vi "AprilTagFieldLayout_New2022.vi"() -> (3 "AprilTagFieldLayout":T1={"AprilTagMap"={}, "FieldLength"=0.0, "FieldWidth"=0.0, "OriginPosition "=enum."kBlueAllianceWallRightSide,", "OriginPose3d"={"Translation3d"={"X"=0.0, "Y"=0.0, "Z"=0.0}, "Rotation3d"={"Q_quaternion"={"R"=1.0, "V"=[0.0, 0.0, 0.0]}}}} {"OriginPose3d"."Translation3d"."Z" format="%14.3f"; "OriginPose3d"."Translation3d"."Y" format="%14.3f"; "OriginPose3d"."Translation3d"."X" format="%14.3f"})   [LabVIEW 2019, in "Trajectory_Library.lvlib"]
doc: "Define the FRC 2022 April Tag field layout.\n\nNOTE -- This function has not been completed.\n\nInputs:\n <none>\n\nOutputs:\n -- AprilTagFieldLayout -- AprilTagFieldLayout -- Data cluster containing field definition."
uses:
  Trajectory_Library.lvlib
  TypeDef/AprilTagFieldLayout.ctl
  TypeDef/AprilTag.ctl
  TypeDef/POSE3D.ctl
  TypeDef/TRANSLATION3D.ctl
  TypeDef/ROTATION3D.ctl
  TypeDef/QUATERNION.ctl
  Enum/AprilTagFieldLayoutOrignPosition_ENUM.ctl
  AprilTag_GetAll.vi
  Quaternion_Normalize.vi
  Quaternion_New_Default.vi
panel:
  # "NOT DONE"
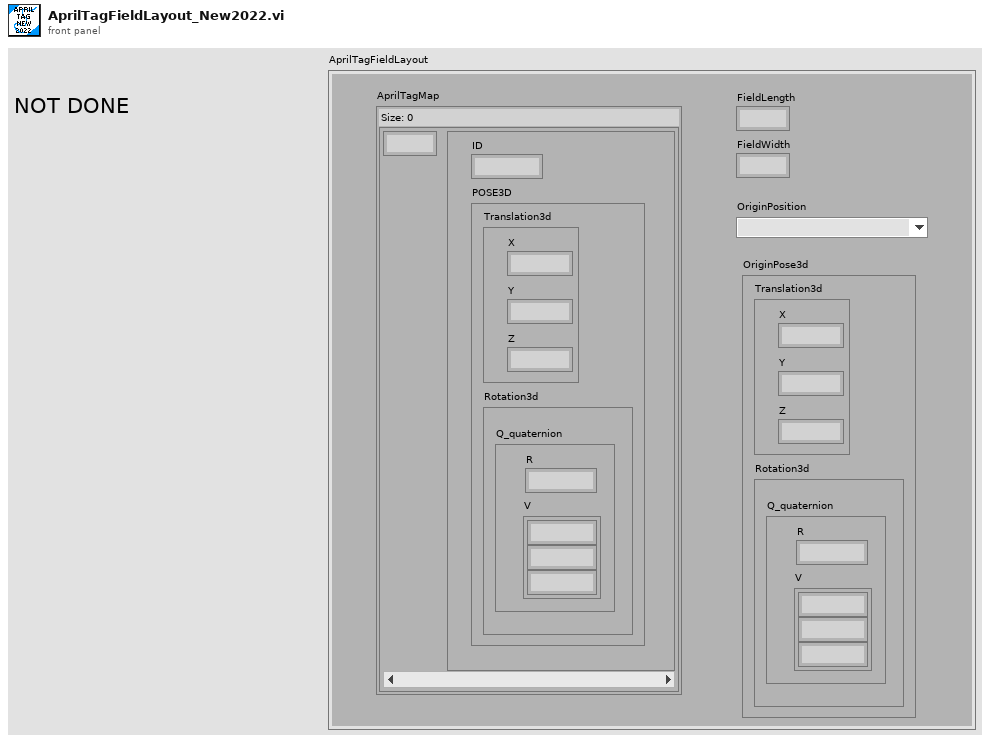
[diagram p1: front panel]
types:
  T1 = typedef "Trajectory_Library.lvlib/AprilTagFieldLayout.ctl" = cluster{"AprilTagMap":map{i32, T2}, "FieldLength":dbl, "FieldWidth":dbl, "OriginPosition ":T7, "OriginPose3d":T3}
  T2 = typedef "Trajectory_Library.lvlib/AprilTag.ctl" = cluster{"ID":i32, "POSE3D":T3}
  T3 = typedef "Trajectory_Library.lvlib/POSE3D.ctl" = cluster{"Translation3d":T4, "Rotation3d":T5}
  T4 = typedef "Trajectory_Library.lvlib/TRANSLATION3D.ctl" = cluster{"X":dbl, "Y":dbl, "Z":dbl}
  T5 = typedef "Trajectory_Library.lvlib/ROTATION3D.ctl" = cluster{"Q_quaternion":T6}
  T6 = typedef "Trajectory_Library.lvlib/QUATERNION.ctl" = cluster{"R":dbl, "V":dbl[]}
  T7 = typedef "Trajectory_Library.lvlib/AprilTagFieldLayoutOrignPosition_ENUM.ctl" = enum16{"kBlueAllianceWallRightSide,", "kRedAllianceWallRightSide,"}
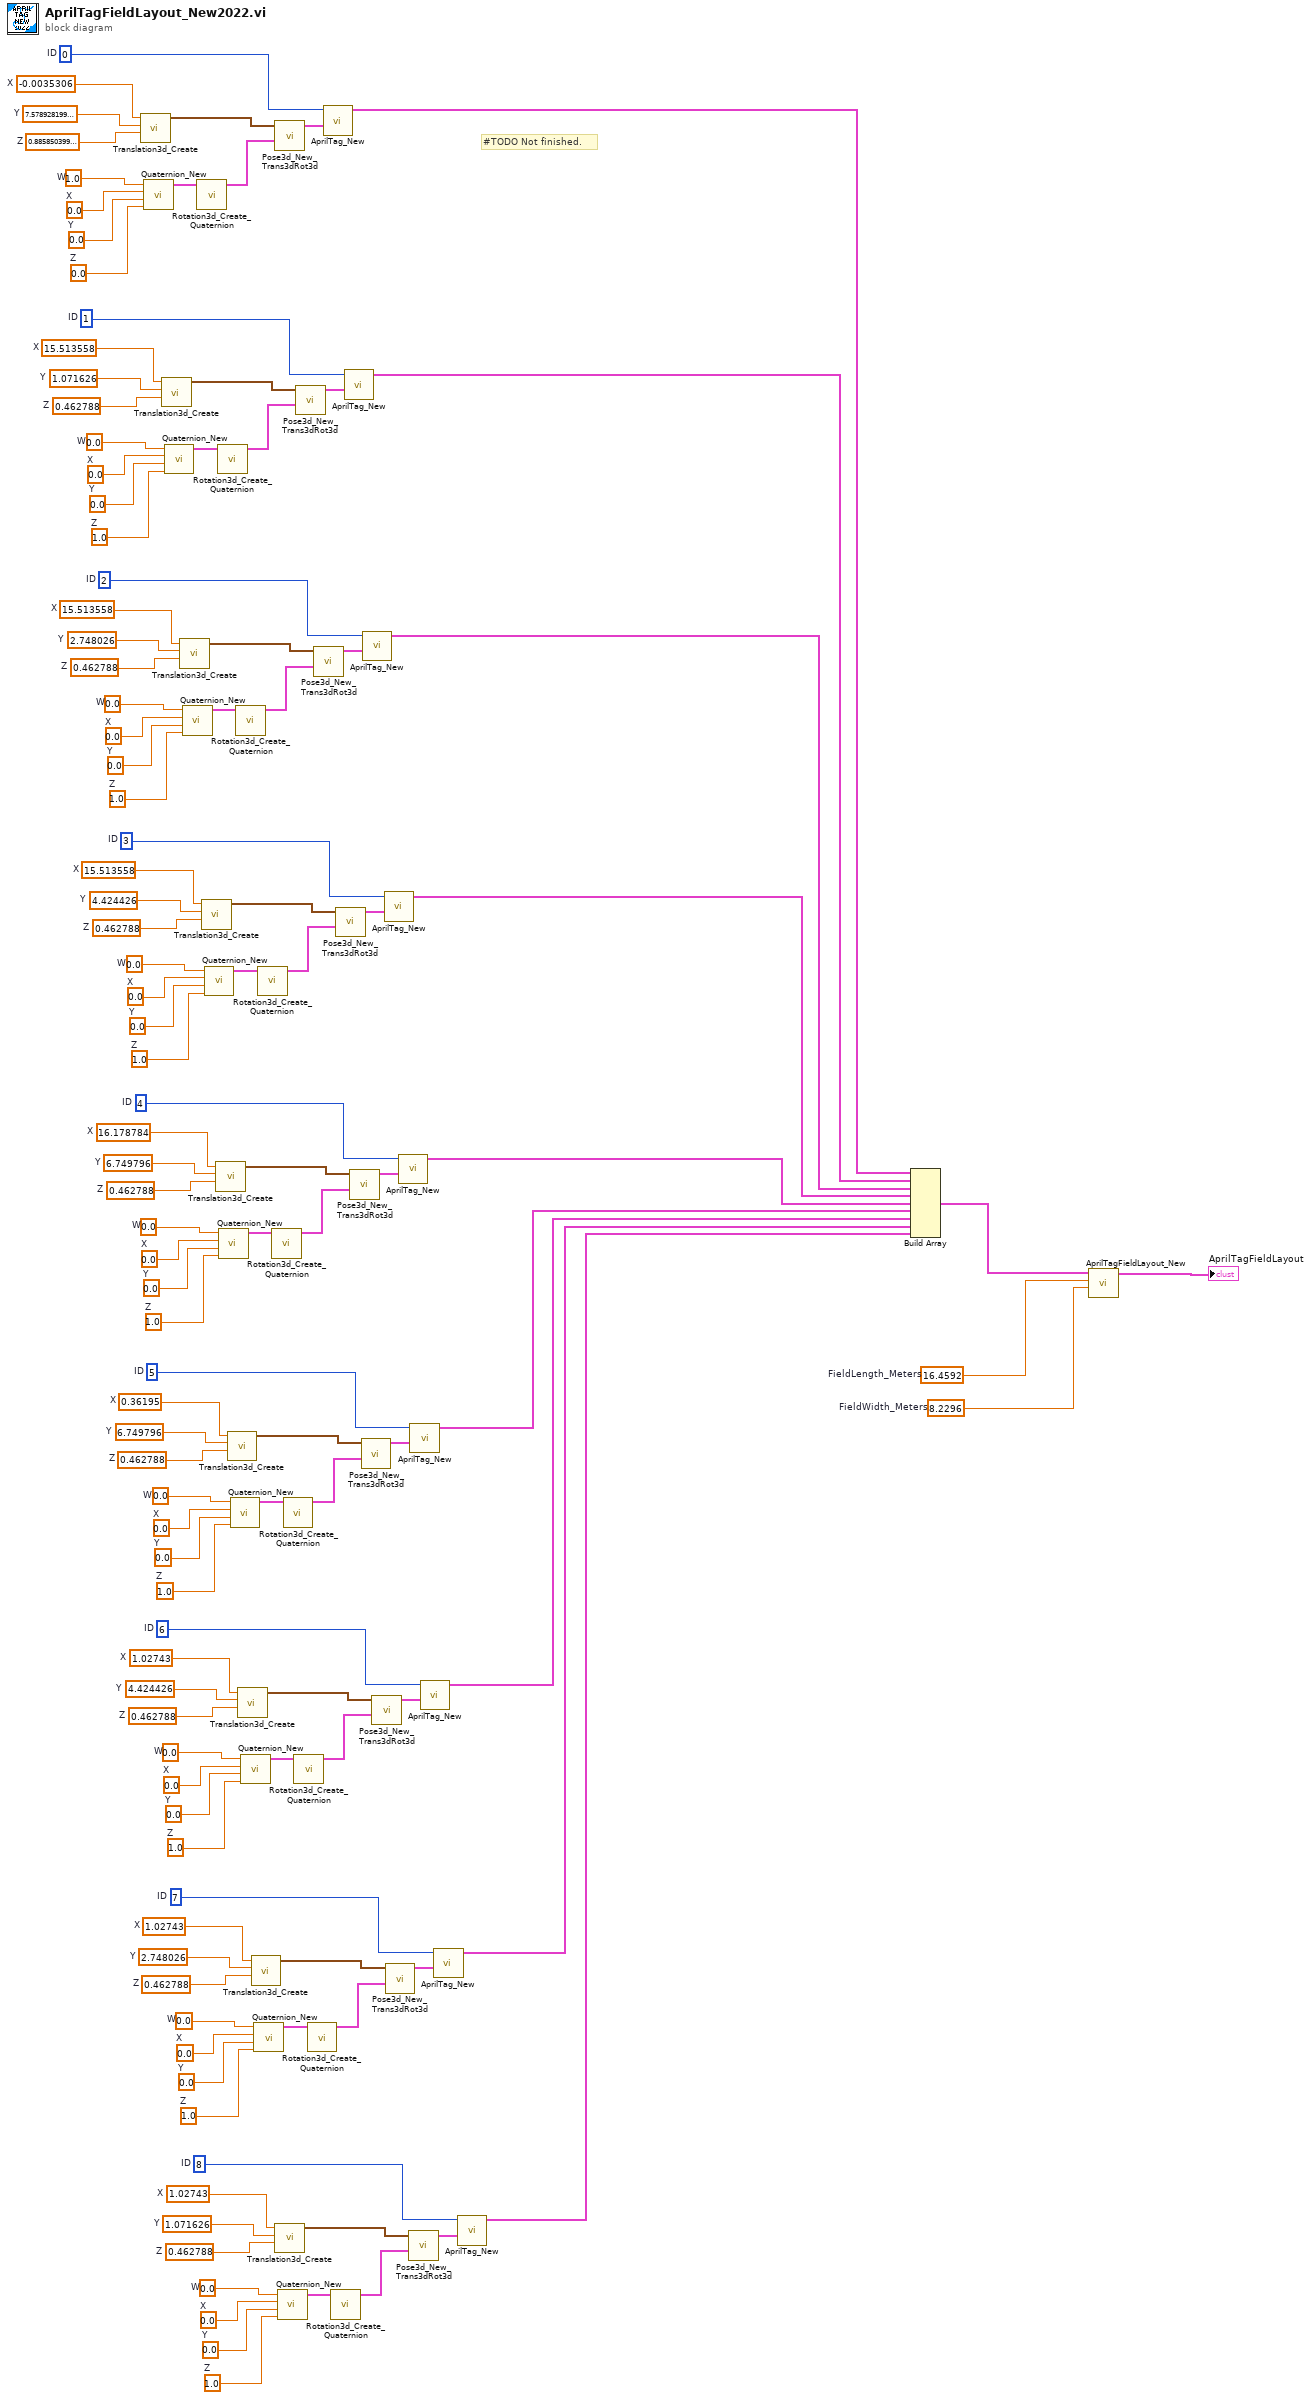
[diagram p0: block diagram]
diagram:
  w3 = 0  # ID
  w5 = -0.0035306  # X
  w6 = 7.578928199999999  # Y
  w7 = 0.8858503999999999  # Z
  w4 = 1.0  # W
  w8 = 0.0  # X
  w9 = 0.0  # Y
  w10 = 0.0  # Z
  w25 = 8  # ID
  w27 = 1.02743  # X
  w28 = 1.071626  # Y
  w29 = 0.462788  # Z
  w26 = 0.0  # W
  w30 = 0.0  # X
  w31 = 0.0  # Y
  w32 = 1.0  # Z
  w37 = 7  # ID
  w39 = 1.02743  # X
  w40 = 2.748026  # Y
  w41 = 0.462788  # Z
  w38 = 0.0  # W
  w42 = 0.0  # X
  w43 = 0.0  # Y
  w44 = 1.0  # Z
  w49 = 6  # ID
  w51 = 1.02743  # X
  w52 = 4.424426  # Y
  w53 = 0.462788  # Z
  w50 = 0.0  # W
  w54 = 0.0  # X
  w55 = 0.0  # Y
  w56 = 1.0  # Z
  w61 = 5  # ID
  w63 = 0.36195  # X
  w64 = 6.749796  # Y
  w65 = 0.462788  # Z
  w62 = 0.0  # W
  w66 = 0.0  # X
  w67 = 0.0  # Y
  w68 = 1.0  # Z
  w73 = 4  # ID
  w75 = 16.178784  # X
  w76 = 6.749796  # Y
  w77 = 0.462788  # Z
  w74 = 0.0  # W
  w78 = 0.0  # X
  w79 = 0.0  # Y
  w80 = 1.0  # Z
  w85 = 3  # ID
  w87 = 15.513558  # X
  w88 = 4.424426  # Y
  w89 = 0.462788  # Z
  w86 = 0.0  # W
  w90 = 0.0  # X
  w91 = 0.0  # Y
  w92 = 1.0  # Z
  w97 = 2  # ID
  w99 = 15.513558  # X
  w100 = 2.748026  # Y
  w101 = 0.462788  # Z
  w98 = 0.0  # W
  w102 = 0.0  # X
  w103 = 0.0  # Y
  w104 = 1.0  # Z
  w109 = 1  # ID
  w111 = 15.513558  # X
  w112 = 1.071626  # Y
  w113 = 0.462788  # Z
  w110 = 0.0  # W
  w114 = 0.0  # X
  w115 = 0.0  # Y
  w116 = 1.0  # Z
  w120 = 8.2296  # FieldWidth_Meters
  w121 = 16.4592  # FieldLength_Meters
  # "#TODO Not finished."
  n1 = call "Translation3d_Create.vi"("Z"=w7, "Y"=w6, "X"=w5) -> ("TRANSLATION3D"=w13:T4)  [unwired: 8 in]
  n2 = call "Quaternion_New.vi"("Z"=w10, "Y"=w9, "X"=w8, "W"=w4) -> ("out Quaternion"=w11:T6)  [unwired: 7 in]
  n3 = call "Translation3d_Create.vi"("Z"=w113, "Y"=w112, "X"=w111) -> ("TRANSLATION3D"=w119:T4)  [unwired: 8 in]
  n4 = call "Quaternion_New.vi"("Z"=w116, "Y"=w115, "X"=w114, "W"=w110) -> ("out Quaternion"=w117:T6)  [unwired: 7 in]
  n5 = call "Translation3d_Create.vi"("Z"=w101, "Y"=w100, "X"=w99) -> ("TRANSLATION3D"=w107:T4)  [unwired: 8 in]
  n6 = call "Quaternion_New.vi"("Z"=w104, "Y"=w103, "X"=w102, "W"=w98) -> ("out Quaternion"=w105:T6)  [unwired: 7 in]
  n7 = call "Rotation3d_Create_Quaternion.vi"("Quaternion"=w11) -> ("Rotation3d"=w12:T5)  [unwired: 10 in]
  n8 = call "Translation3d_Create.vi"("Z"=w89, "Y"=w88, "X"=w87) -> ("TRANSLATION3D"=w95:T4)  [unwired: 8 in]
  n9 = call "Quaternion_New.vi"("Z"=w92, "Y"=w91, "X"=w90, "W"=w86) -> ("out Quaternion"=w93:T6)  [unwired: 7 in]
  n10 = call "Translation3d_Create.vi"("Z"=w77, "Y"=w76, "X"=w75) -> ("TRANSLATION3D"=w83:T4)  [unwired: 8 in]
  n11 = call "Rotation3d_Create_Quaternion.vi"("Quaternion"=w117) -> ("Rotation3d"=w118:T5)  [unwired: 10 in]
  n12 = call "Quaternion_New.vi"("Z"=w80, "Y"=w79, "X"=w78, "W"=w74) -> ("out Quaternion"=w81:T6)  [unwired: 7 in]
  n13 = call "Translation3d_Create.vi"("Z"=w65, "Y"=w64, "X"=w63) -> ("TRANSLATION3D"=w71:T4)  [unwired: 8 in]
  n14 = call "Quaternion_New.vi"("Z"=w68, "Y"=w67, "X"=w66, "W"=w62) -> ("out Quaternion"=w69:T6)  [unwired: 7 in]
  n15 = call "Rotation3d_Create_Quaternion.vi"("Quaternion"=w105) -> ("Rotation3d"=w106:T5)  [unwired: 10 in]
  n16 = call "Translation3d_Create.vi"("Z"=w53, "Y"=w52, "X"=w51) -> ("TRANSLATION3D"=w59:T4)  [unwired: 8 in]
  n17 = call "Quaternion_New.vi"("Z"=w56, "Y"=w55, "X"=w54, "W"=w50) -> ("out Quaternion"=w57:T6)  [unwired: 7 in]
  n18 = call "Translation3d_Create.vi"("Z"=w41, "Y"=w40, "X"=w39) -> ("TRANSLATION3D"=w47:T4)  [unwired: 8 in]
  n19 = call "Quaternion_New.vi"("Z"=w44, "Y"=w43, "X"=w42, "W"=w38) -> ("out Quaternion"=w45:T6)  [unwired: 7 in]
  n20 = call "Rotation3d_Create_Quaternion.vi"("Quaternion"=w93) -> ("Rotation3d"=w94:T5)  [unwired: 10 in]
  n21 = call "Rotation3d_Create_Quaternion.vi"("Quaternion"=w81) -> ("Rotation3d"=w82:T5)  [unwired: 10 in]
  n22 = call "Pose3d_New_Trans3dRot3d.vi"("Rotation3d"=w12, "Translation3d"=w13) -> ("outPose3d"=w2:T3)  [unwired: 9 in]
  n23 = call "Translation3d_Create.vi"("Z"=w29, "Y"=w28, "X"=w27) -> ("TRANSLATION3D"=w35:T4)  [unwired: 8 in]
  n24 = call "Quaternion_New.vi"("Z"=w32, "Y"=w31, "X"=w30, "W"=w26) -> ("out Quaternion"=w33:T6)  [unwired: 7 in]
  n25 = call "Rotation3d_Create_Quaternion.vi"("Quaternion"=w69) -> ("Rotation3d"=w70:T5)  [unwired: 10 in]
  n26 = call "Rotation3d_Create_Quaternion.vi"("Quaternion"=w57) -> ("Rotation3d"=w58:T5)  [unwired: 10 in]
  n27 = call "Pose3d_New_Trans3dRot3d.vi"("Rotation3d"=w118, "Translation3d"=w119) -> ("outPose3d"=w108:T3)  [unwired: 9 in]
  n28 = call "Rotation3d_Create_Quaternion.vi"("Quaternion"=w45) -> ("Rotation3d"=w46:T5)  [unwired: 10 in]
  n29 = call "Pose3d_New_Trans3dRot3d.vi"("Rotation3d"=w106, "Translation3d"=w107) -> ("outPose3d"=w96:T3)  [unwired: 9 in]
  n30 = call "AprilTag_New.vi"("POSE3D"=w2, "ID"=w3) -> ("AprilTag"=w1:T2)  [unwired: 9 in]
  n31 = call "Rotation3d_Create_Quaternion.vi"("Quaternion"=w33) -> ("Rotation3d"=w34:T5)  [unwired: 10 in]
  n32 = call "Pose3d_New_Trans3dRot3d.vi"("Rotation3d"=w94, "Translation3d"=w95) -> ("outPose3d"=w84:T3)  [unwired: 9 in]
  n33 = call "AprilTag_New.vi"("POSE3D"=w108, "ID"=w109) -> ("AprilTag"=w22:T2)  [unwired: 9 in]
  n34 = call "Pose3d_New_Trans3dRot3d.vi"("Rotation3d"=w82, "Translation3d"=w83) -> ("outPose3d"=w72:T3)  [unwired: 9 in]
  n35 = call "Pose3d_New_Trans3dRot3d.vi"("Rotation3d"=w70, "Translation3d"=w71) -> ("outPose3d"=w60:T3)  [unwired: 9 in]
  n36 = call "AprilTag_New.vi"("POSE3D"=w96, "ID"=w97) -> ("AprilTag"=w21:T2)  [unwired: 9 in]
  n37 = call "Pose3d_New_Trans3dRot3d.vi"("Rotation3d"=w58, "Translation3d"=w59) -> ("outPose3d"=w48:T3)  [unwired: 9 in]
  n38 = call "AprilTag_New.vi"("POSE3D"=w84, "ID"=w85) -> ("AprilTag"=w20:T2)  [unwired: 9 in]
  n39 = call "Pose3d_New_Trans3dRot3d.vi"("Rotation3d"=w46, "Translation3d"=w47) -> ("outPose3d"=w36:T3)  [unwired: 9 in]
  n40 = call "AprilTag_New.vi"("POSE3D"=w72, "ID"=w73) -> ("AprilTag"=w19:T2)  [unwired: 9 in]
  n41 = call "Pose3d_New_Trans3dRot3d.vi"("Rotation3d"=w34, "Translation3d"=w35) -> ("outPose3d"=w24:T3)  [unwired: 9 in]
  n42 = call "AprilTag_New.vi"("POSE3D"=w60, "ID"=w61) -> ("AprilTag"=w18:T2)  [unwired: 9 in]
  n43 = call "AprilTag_New.vi"("POSE3D"=w48, "ID"=w49) -> ("AprilTag"=w17:T2)  [unwired: 9 in]
  n44 = call "AprilTag_New.vi"("POSE3D"=w36, "ID"=w37) -> ("AprilTag"=w16:T2)  [unwired: 9 in]
  n45 = call "AprilTag_New.vi"("POSE3D"=w24, "ID"=w25) -> ("AprilTag"=w15:T2)  [unwired: 9 in]
  n46 = Build Array(w1, w22, w21, w20, w19, w18, w17, w16, w15) -> (w23:T2[])
  n47 = call "AprilTagFieldLayout_New.vi"("FieldWidth_Meters"=w120, "FieldLength_Meters"=w121, "AprilTags"=w23) -> ("AprilTagFieldLayout"=→"AprilTagFieldLayout":T1)  [unwired: 8 in]
